vi "stage_init.vi"(11 "stage init settings":T2={"piezo_activeX_references"={" piezo_x"=refnum, "piezo_y"=refnum, " piezo_z"=refnum}, "stepper_activeX_references"={"MG17Motor x"=refnum, "MG17Motor y"=refnum, "MG17Motor z"=refnum}, "piezo serial numbers"={"x-axis"=91897094, "y_axis"=91897095, "z_axis"=91897096}, "stepper serial numbers"={"x-axis"=90897056, "y_axis"=90897057, "z_axis"=90897058}, "stepper_parameters"="dha_apt_stepper"}) -> (0 "error out":errorcluster, 3 "Stage reference":T1)   [LabVIEW 2018]
uses:
  stage_init_type.ctl
  stage_reference_type.ctl
  <userlib>/stepper/velocity settings.ctl
  <userlib>/stepper/travel limits.ctl
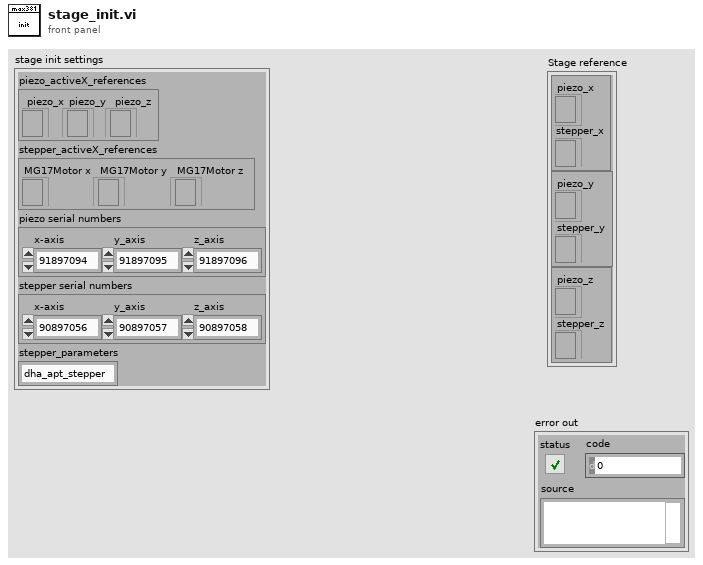
[diagram p1: front panel]
types:
  T1 = typedef "stage_reference_type.ctl" = cluster{cluster{"piezo_x":refnum<k7>, "stepper_x":refnum<k7>}, cluster{"piezo_y":refnum<k7>, "stepper_y":refnum<k7>}, cluster{"piezo_z":refnum<k7>, "stepper_z":refnum<k7>}}
  T2 = typedef "stage_init_type.ctl" = cluster{"piezo_activeX_references":cluster{" piezo_x":refnum<k7>, "piezo_y":refnum<k7>, " piezo_z":refnum<k7>}, "stepper_activeX_references":cluster{"MG17Motor x":refnum<k7>, "MG17Motor y":refnum<k7>, "MG17Motor z":refnum<k7>}, "piezo serial numbers":cluster{"x-axis":i32, "y_axis":i32, "z_axis":i32}, "stepper serial numbers":cluster{"x-axis":i32, "y_axis":i32, "z_axis":i32}, "stepper_parameters":string}
  T3 = typedef "travel limits.ctl" = cluster{"pfRevPosLimit":sgl, "pfFwdPosLimit":sgl, "plLimitMode":i32}
  T4 = typedef "velocity settings.ctl" = cluster{"pfMinVel":sgl, "pfAccn":sgl, "pfMaxVel":sgl}
  T5 = cluster{" piezo_x":refnum<k7>, "piezo_y":refnum<k7>, " piezo_z":refnum<k7>}
  T6 = cluster{"MG17Motor x":refnum<k7>, "MG17Motor y":refnum<k7>, "MG17Motor z":refnum<k7>}
  T7 = cluster{"x-axis":i32, "y_axis":i32, "z_axis":i32}
  T8 = cluster{"reference out":refnum<k7>, "reference out":refnum<k7>}
  T9 = cluster{cluster{"reference out":refnum<k7>, "reference out":refnum<k7>}, cluster{"reference out":refnum<k7>, "reference out":refnum<k7>}, cluster{"reference out":refnum<k7>, "reference out":refnum<k7>}}
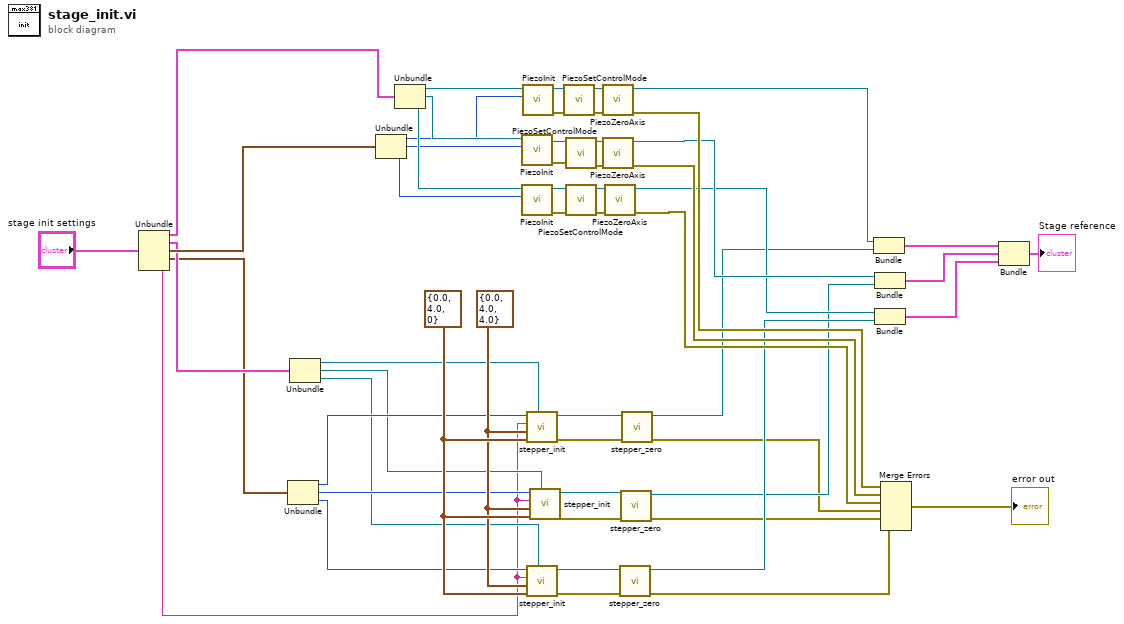
[diagram p0: block diagram]
diagram:
  w49 = T3 {"pfRevPosLimit"=0.0, "pfFwdPosLimit"=4.0, "plLimitMode"=0} ("travel limits")
  w48 = T4 {"pfMinVel"=0.0, "pfAccn"=4.0, "pfMaxVel"=4.0} ("velocity parameters")
  n1 = Unbundle("stage init settings") -> ("piezo_activeX_references"=w22:T5, "stepper_activeX_references"=w20:T6, "piezo serial numbers"=w21:T7, "stepper serial numbers"=w19:T7, "stepper_parameters"=w18:string)
  n2 = Unbundle(w19) -> ("x-axis"=w29:i32, "y_axis"=w28:i32, "z_axis"=w27:i32)
  n3 = Unbundle(w20) -> ("MG17Motor x"=w26:refnum<k7>, "MG17Motor y"=w25:refnum<k7>, "MG17Motor z"=w24:refnum<k7>)
  n4 = Unbundle(w21) -> ("x-axis"=w32:i32, "y_axis"=w31:i32, "z_axis"=w30:i32)
  n5 = Unbundle(w22) -> ("piezo_x"=w35:refnum<k7>, "piezo_y"=w34:refnum<k7>, "piezo_z"=w33:refnum<k7>)
  n6 = call <userlib>:"PiezoInit.vi"("reference"=w34, "HWSerialNum"=w31) -> ("reference out"=w52:refnum<k7>, "error out"=w54:errorcluster)  [unwired: 7 in]
  n7 = call <userlib>:"PiezoInit.vi"("reference"=w33, "HWSerialNum"=w30) -> ("reference out"=w51:refnum<k7>, "error out"=w55:errorcluster)  [unwired: 7 in]
  n8 = call <userlib>:"PiezoInit.vi"("reference"=w35, "HWSerialNum"=w32) -> ("reference out"=w50:refnum<k7>, "error out"=w53:errorcluster)  [unwired: 7 in]
  n9 = call <userlib>:"stepper_init.vi"("MG17Motor"=w26, "travel limits"=w49, "velocity parameters"=w48, "parameter set"=w18, "HWSerialNum"=w29) -> ("error out"=w41:errorcluster, "reference out"=w40:refnum<k7>)  [unwired: 3 in, 2 out]
  n10 = call <userlib>:"stepper_init.vi"("MG17Motor"=w24, "travel limits"=w49, "velocity parameters"=w48, "parameter set"=w18, "HWSerialNum"=w27) -> ("error out"=w36:errorcluster, "reference out"=w37:refnum<k7>)  [unwired: 3 in, 2 out]
  n11 = call <userlib>:"stepper_init.vi"("MG17Motor"=w25, "travel limits"=w49, "velocity parameters"=w48, "parameter set"=w18, "HWSerialNum"=w28) -> ("error out"=w38:errorcluster, "reference out"=w39:refnum<k7>)  [unwired: 3 in, 2 out]
  n12 = call <userlib>:"PiezoSetControlMode.vi"("error in (no error)"=w53, "reference"=w50) -> ("error out"=w47:errorcluster, "reference out"=w46:refnum<k7>)  [unwired: 8 in]
  n13 = call <userlib>:"PiezoSetControlMode.vi"("error in (no error)"=w54, "reference"=w52) -> ("error out"=w44:errorcluster, "reference out"=w45:refnum<k7>)  [unwired: 8 in]
  n14 = call <userlib>:"PiezoSetControlMode.vi"("error in (no error)"=w55, "reference"=w51) -> ("error out"=w42:errorcluster, "reference out"=w43:refnum<k7>)  [unwired: 8 in]
  n15 = call <userlib>:"PiezoZeroAxis.vi"("error in (no error)"=w47, "reference"=w46) -> ("error out"=w12:errorcluster, "reference out"=w11:refnum<k7>)  [unwired: 8 in]
  n16 = call <userlib>:"PiezoZeroAxis.vi"("error in (no error)"=w44, "reference"=w45) -> ("error out"=w9:errorcluster, "reference out"=w10:refnum<k7>)  [unwired: 8 in]
  n17 = call <userlib>:"PiezoZeroAxis.vi"("error in (no error)"=w42, "reference"=w43) -> ("error out"=w7:errorcluster, "reference out"=w8:refnum<k7>)  [unwired: 8 in]
  n18 = call <userlib>:"stepper_zero.vi"("error in (no error)"=w36, "reference"=w37) -> ("error out"=w5:errorcluster, "reference out"=w6:refnum<k7>)  [unwired: 8 in]
  n19 = call <userlib>:"stepper_zero.vi"("error in (no error)"=w38, "reference"=w39) -> ("error out"=w4:errorcluster, "reference out"=w3:refnum<k7>)  [unwired: 8 in]
  n20 = call <userlib>:"stepper_zero.vi"("error in (no error)"=w41, "reference"=w40) -> ("error out"=w2:errorcluster, "reference out"=w1:refnum<k7>)  [unwired: 8 in]
  n21 = Bundle("reference out"=w11, "reference out"=w1) -> (w17:T8)  [unwired: 1 in]
  n22 = Bundle("reference out"=w10, "reference out"=w3) -> (w16:T8)  [unwired: 1 in]
  n23 = Bundle("reference out"=w8, "reference out"=w6) -> (w15:T8)  [unwired: 1 in]
  n24 = Merge Errors(w12, w9, w7, w2, w4, w5) -> (→"error out":errorcluster)
  n25 = Bundle(w17, w16, w15) -> (→"Stage reference":T9)  [unwired: 1 in]
